vi "WriteLastOF.vi"(8 "errin":errorcluster, 11 "OF to save":string) -> (0 "errout":errorcluster)   [LabVIEW 2020]
doc: "Sauvegarde le dernier OF dans le fichier Conf.ini"
uses:
  <vilib>/Utility/config.llb/Write Key (String).vi
  <vilib>/Utility/config.llb/NI_LVConfig.lvlib
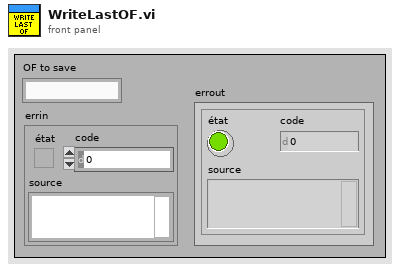
[diagram p1: front panel]
types:
  T1 = typedef "NI_LVConfig.lvlib/Config Data RefNum.ctl" = refnum<k1>
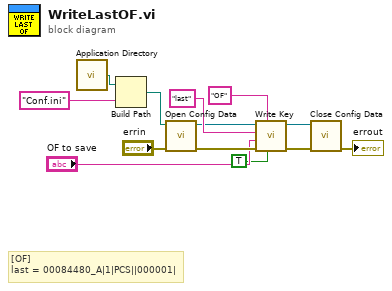
[diagram p0: block diagram]
diagram:
  # "[OF]\nlast = 00084480_A|1|PCS||000001|"
  n1 = call <vilib>:"Application Directory.vi"() -> ("Application Directory"=w7:path)
  n2 = Build Path ("Composer un chemin")(base path=w7, name or relative path="Conf.ini") -> (appended path=w9:path)
  n3 = call <vilib>:"Open Config Data.vi"("error in (no error)"="errin", "configuration file path"=w9) -> ("error out"=w5:errorcluster, "refnum"=w10:T1)  [unwired: 7 in, 1 out]
  n4 = call-poly <vilib>:"Write Key.vi"("write raw string? (F)"=TRUE, "section"="OF", "error in (no error)"=w5, "value"="OF to save", "key"="last", "refnum"=w10) -> ("error out"=w4:errorcluster, "refnum out"=w13:T1)  [unwired: 3 in, 1 out]
  n5 = call <vilib>:"Close Config Data.vi"("error in (no error)"=w4, "refnum"=w13) -> ("error out"=→"errout":errorcluster)  [unwired: 8 in, 1 out]
